vi "Set CAN_Raw.vi"(8 "error in (no error)":errorcluster, 9 "Data":u8[](array[numeric]), 10 "Identifier":u32, 11 "connection info":T1) -> (0 "error out":errorcluster, 2 "Sent?":bool, 3 "connection info":T1)   [LabVIEW 2023, in "J1939 Host Automation API.lvlib"]
uses:
  J1939 Host Automation API.lvlib
  <vilib>/NI/STM/TCP/TCP Connection Info.ctl
  <vilib>/NI/STM/SubVIs/MetaDataElement.ctl
  Addon/Support Libraries/J1939 Utilities/Types/CAN Outgoing Message Cluster.ctl
  Addon/Addon Shared/J1939 Addon Shared.lvlib
  Addon/Support Libraries/J1939 Utilities/J1939 Utilities.lvlib
  <vilib>/NI/STM/NI STM.lvlib
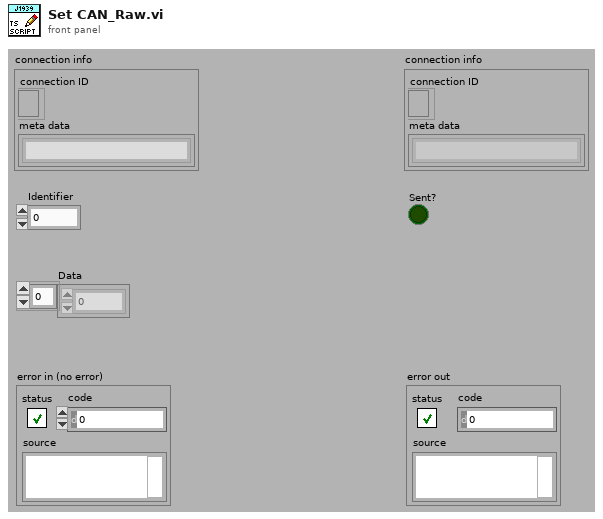
[diagram p1: front panel]
types:
  T1 = typedef "NI STM.lvlib/TCP Connection Info.ctl" = cluster{"connection ID":refnum<k5>, "meta data":T2[]}
  T2 = typedef "NI STM.lvlib/MetaDataElement.ctl" = string
  T3 = typedef "J1939 Utilities.lvlib/CAN Outgoing Message Cluster.ctl" = cluster{"Identifier":u32, "Data":u8[]}
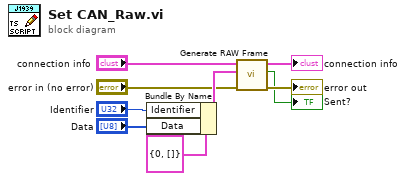
[diagram p0: block diagram]
diagram:
  n1 = Bundle By Name(cluster=T3 {"Identifier"=0, "Data"=[]} ("Data to Send"), "Identifier"="Identifier", "Data"="Data") -> (w6:T3)
  n2 = call "Generate RAW Frame.vi"("error in (no error)"="error in (no error)", "Data to Send"=w6, "connection info"="connection info") -> ("error out"=→"error out":errorcluster, "Sent?"=→"Sent?":bool, "connection info"=→"connection info":T1)  [unwired: 6 in]
